vi "Signalgenerator (2).vi"() -> ()   [LabVIEW 2013]
panel:
  in  "Set Phase":bool
  in  "Phase":dbl
  in  "Set Offset":bool
  in  "Offset":dbl
  in  "Set Amplitude":bool
  in  "Amplitude":dbl
  in  "Set Frequency":bool
  in  "Frequency":dbl
  in  "Waveform":T1(radio)
  in  "Display Mode":T2(radio)
  in  "Read":bool
  in  "Write":bool
  in  "Exit":bool
  in  "Connect":bool
  in  "VISA Address":refnum<visa-resource-name>
  out "Return":string
  in  "Command":string
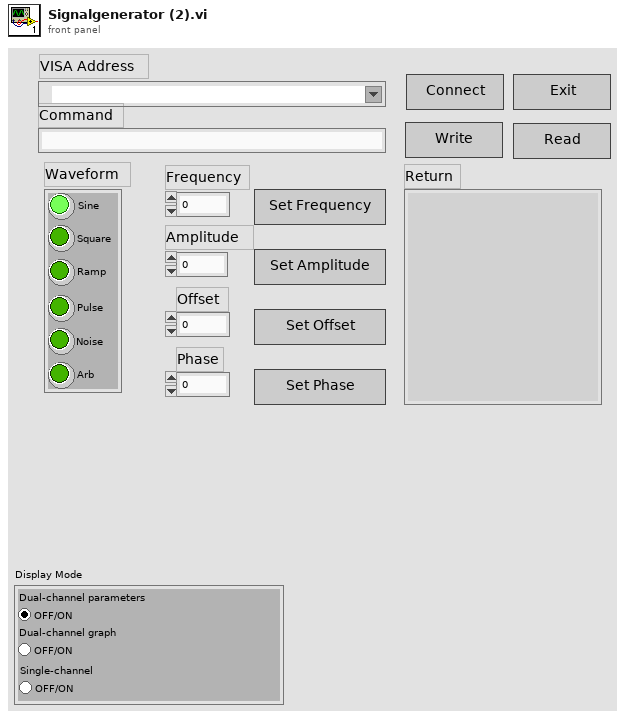
[diagram p1: front panel]
types:
  T1 = enum32{"Sine", "Square", "Ramp", "Pulse", "Noise", "Arb"}
  T2 = enum32{"Dual-channel parameters", "Dual-channel graph", "Single-channel"}
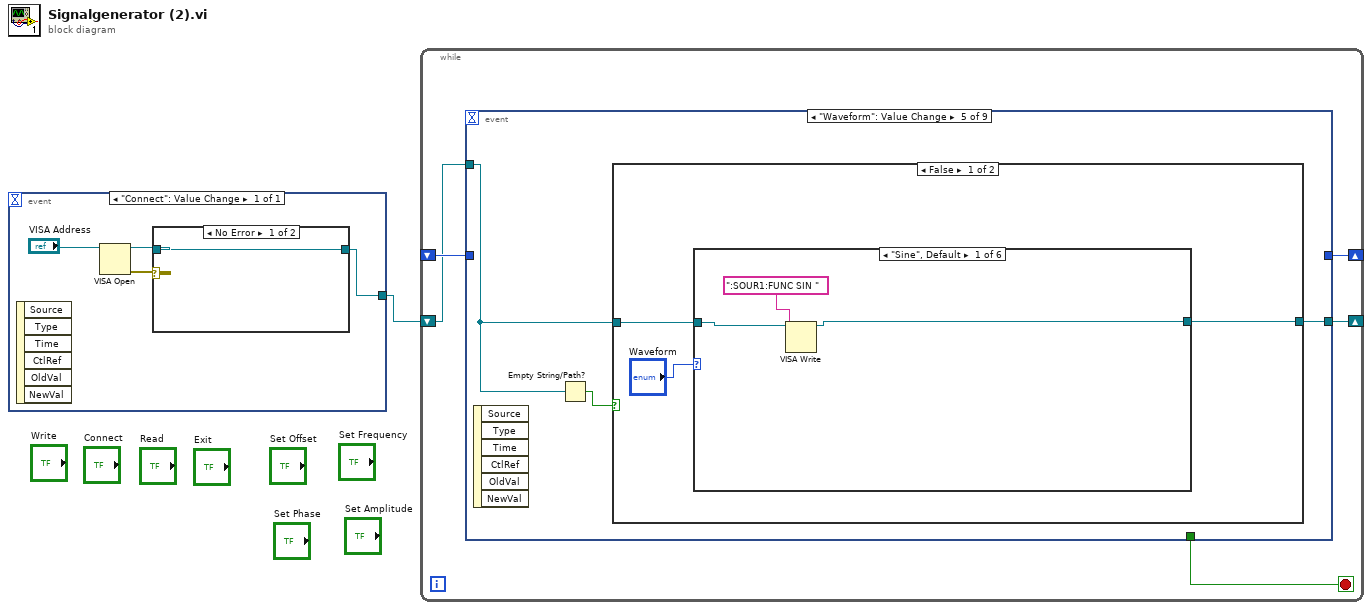
[diagram p0: block diagram]
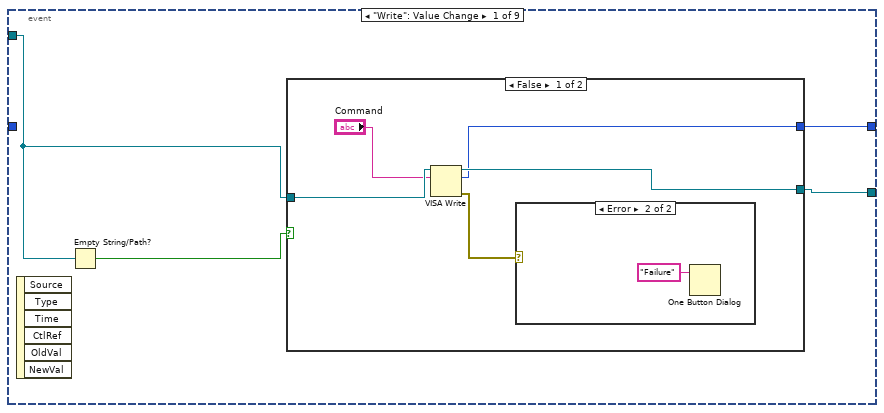
[diagram p2: hidden frame]
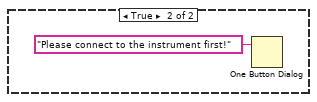
[diagram p4: hidden frame]
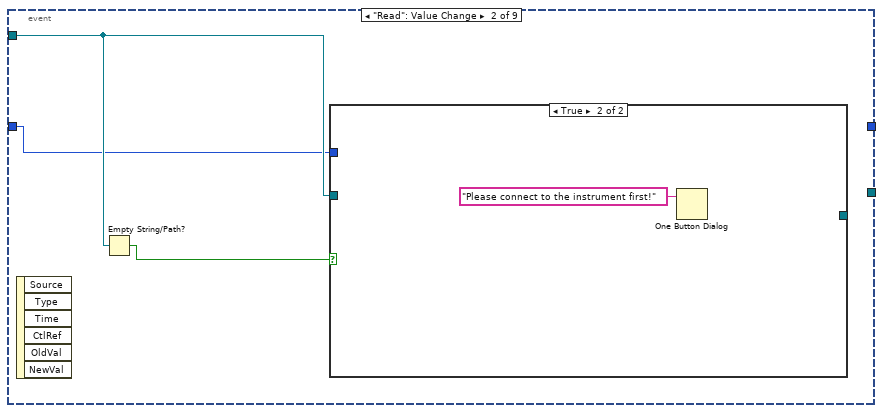
[diagram p5: hidden frame]
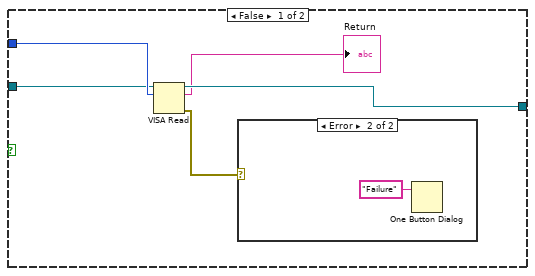
[diagram p6: hidden frame]
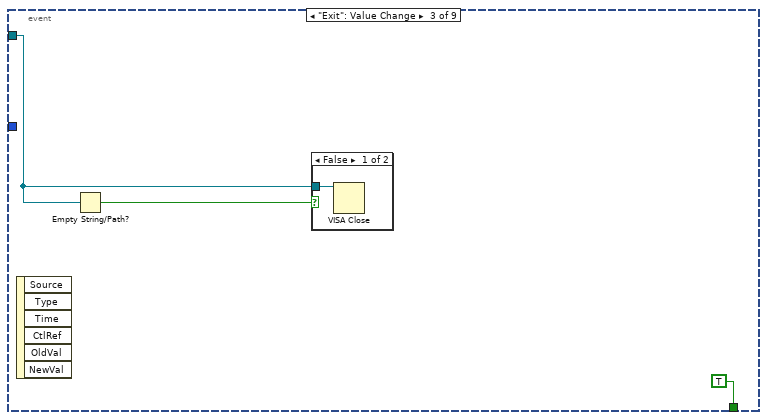
[diagram p8: hidden frame]
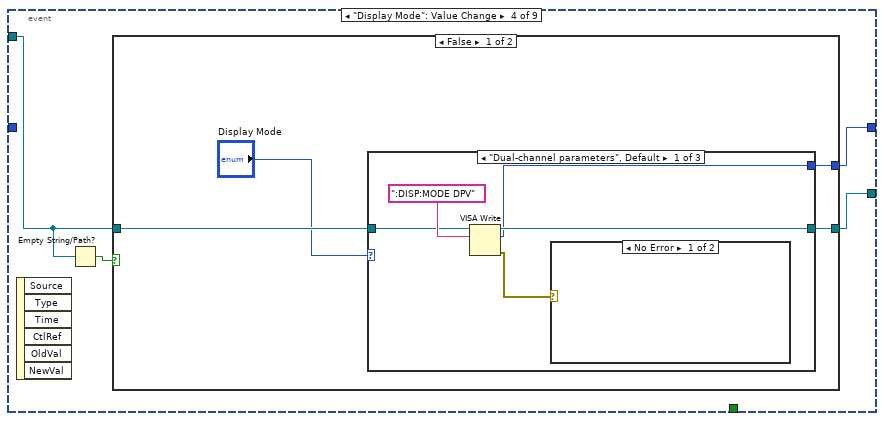
[diagram p10: hidden frame]
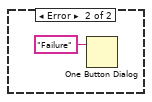
[diagram p11: hidden frame]
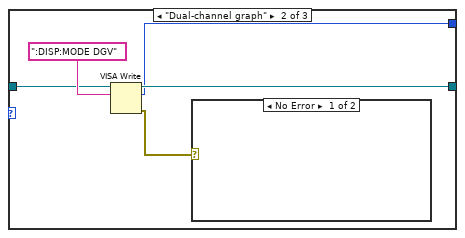
[diagram p12: hidden frame]
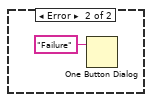
[diagram p13: hidden frame]
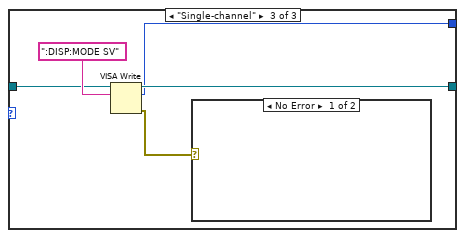
[diagram p14: hidden frame]
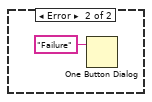
[diagram p15: hidden frame]
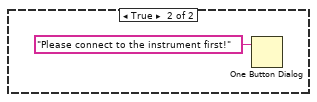
[diagram p16: hidden frame]
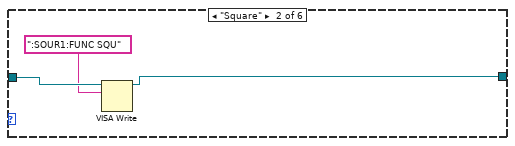
[diagram p17: hidden frame]
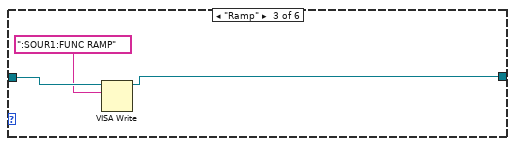
[diagram p18: hidden frame]
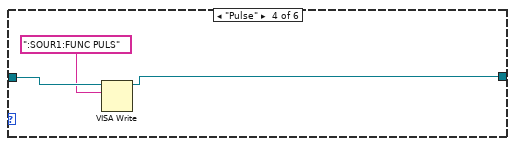
[diagram p19: hidden frame]
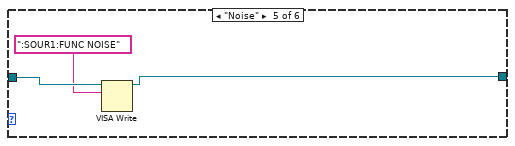
[diagram p20: hidden frame]
diagram:
  n1 = event shown="[0] \"Connect\": Value Change" {
    selector: _ -> [_]
    dyn-events: _ -> [_]
    timeout: _ -> [_]
    tunnel: [w3] -> w1
    event "Connect": Value Change {
      n2 = event-data() -> ()  [unwired: 1 in, 6 out]
      n3 = VISA Open(VISA resource name="VISA Address") -> (VISA resource name=w4:refnum<visa-resource-name>, error out=w5:errorcluster)  [unwired: 4 in]
      n4 = case shown="No Error" w5 {
        tunnel: w4 -> [w6 _]
        tunnel: [w6 _] -> w3
        frame No Error {
        }
        frame Error {
          n5 = One Button Dialog(message="Connect failed!\nInvalid address!") -> ()  [unwired: 1 in, 1 out]
        }
      }
    }
  }
  n6 = while {
    shift-right: [w10] -> _
    shift-left: w1 -> [w11]
    shift-right: [w9] -> _
    shift-left: _ -> [w12]
    stop <- w8 stop-if-true
    n7 = event shown="[4] \"Waveform\": Value Change" {
      selector: _ -> [_ _ _ _ _ _ _ _ _]
      dyn-events: _ -> [_ _ _ _ _ _ _ _ _]
      timeout: _ -> [_ _ _ _ _ _ _ _ _]
      tunnel: w12 -> [_ w24 _ _ _ _ _ _ _]
      tunnel: w11 -> [w15 w25 w35 w38 w66 w92 w105 w120 w134]
      tunnel: [w14 _ _ w40 w65 w90 w103 w117 w131] -> w10
      tunnel: [w13 _ _ w41 _ w91 w104 w118 w132] -> w9
      tunnel: [_ _ TRUE _ _ _ _ _ _] -> w8
      event "Write": Value Change {
        n8 = event-data() -> ()  [unwired: 1 in, 6 out]
        n9 = Empty String/Path?(string/path=w15) -> (empty?=w16:bool)
        n10 = case shown="False" w16 {
          tunnel: [w20 _] -> w14
          tunnel: [w19 _] -> w13
          tunnel: w15 -> [w18 _]
          frame False {
            n11 = VISA Write(VISA resource name=w18, write buffer="Command") -> (VISA resource name out=w20:refnum<visa-resource-name>, return count=w19:u32, error out=w21:errorcluster)  [unwired: 1 in]
            n12 = case shown="Error" w21 {
              frame No Error {
              }
              frame Error {
                n13 = One Button Dialog(message="Failure") -> ()  [unwired: 1 in, 1 out]
              }
            }
          }
          frame True {
            n14 = One Button Dialog(message="Please connect to the instrument first!") -> ()  [unwired: 1 in, 1 out]
          }
        }
      }
      event "Read": Value Change {
        n15 = event-data() -> ()  [unwired: 1 in, 6 out]
        n16 = Empty String/Path?(string/path=w25) -> (empty?=w26:bool)
        n17 = case shown="True" w26 {
          tunnel: [w31 _] -> _
          tunnel: w24 -> [w29 _]
          tunnel: w25 -> [w28 _]
          frame False {
            n18 = VISA Read(VISA resource name=w28, byte count=w29) -> (VISA resource name out=w31:refnum<visa-resource-name>, read buffer=→"Return":string, error out=w30:errorcluster)  [unwired: 1 in, 1 out]
            n19 = case shown="Error" w30 {
              frame No Error {
              }
              frame Error {
                n20 = One Button Dialog(message="Failure") -> ()  [unwired: 1 in, 1 out]
              }
            }
          }
          frame True {
            n21 = One Button Dialog(message="Please connect to the instrument first!") -> ()  [unwired: 1 in, 1 out]
          }
        }
      }
      event "Exit": Value Change {
        n22 = event-data() -> ()  [unwired: 1 in, 6 out]
        n23 = Empty String/Path?(string/path=w35) -> (empty?=w36:bool)
        n24 = case shown="False" w36 {
          tunnel: w35 -> [w37 _]
          frame False {
            n25 = VISA Close(VISA resource name=w37) -> ()  [unwired: 1 in, 1 out]
          }
          frame True {
          }
        }
      }
      event "Display Mode": Value Change {
        n26 = event-data() -> ()  [unwired: 1 in, 6 out]
        n27 = Empty String/Path?(string/path=w38) -> (empty?=w39:bool)
        n28 = case shown="False" w39 {
          tunnel: [w45 _] -> w40
          tunnel: [w44 _] -> w41
          tunnel: w38 -> [w43 _]
          frame False {
            n29 = case shown="\"Dual-channel parameters\", Default" "Display Mode" {
              tunnel: [w48 w54 w60] -> w45
              tunnel: [w47 w53 w59] -> w44
              tunnel: w43 -> [w46 w52 w58]
              frame "Dual-channel parameters", Default {
                n30 = VISA Write(VISA resource name=w46, write buffer=":DISP:MODE DPV" ("Command 2")) -> (VISA resource name out=w48:refnum<visa-resource-name>, return count=w47:u32, error out=w49:errorcluster)  [unwired: 1 in]
                n31 = case shown="No Error" w49 {
                  frame No Error {
                  }
                  frame Error {
                    n32 = One Button Dialog(message="Failure") -> ()  [unwired: 1 in, 1 out]
                  }
                }
              }
              frame "Dual-channel graph" {
                n33 = VISA Write(VISA resource name=w52, write buffer=":DISP:MODE DGV" ("Command 2")) -> (VISA resource name out=w54:refnum<visa-resource-name>, return count=w53:u32, error out=w55:errorcluster)  [unwired: 1 in]
                n34 = case shown="No Error" w55 {
                  frame No Error {
                  }
                  frame Error {
                    n35 = One Button Dialog(message="Failure") -> ()  [unwired: 1 in, 1 out]
                  }
                }
              }
              frame "Single-channel" {
                n36 = VISA Write(VISA resource name=w58, write buffer=":DISP:MODE SV" ("Command 2")) -> (VISA resource name out=w60:refnum<visa-resource-name>, return count=w59:u32, error out=w61:errorcluster)  [unwired: 1 in]
                n37 = case shown="No Error" w61 {
                  frame No Error {
                  }
                  frame Error {
                    n38 = One Button Dialog(message="Failure") -> ()  [unwired: 1 in, 1 out]
                  }
                }
              }
            }
          }
          frame True {
            n39 = One Button Dialog(message="Please connect to the instrument first!") -> ()  [unwired: 1 in, 1 out]
          }
        }
      }
      event "Waveform": Value Change {
        n40 = event-data() -> ()  [unwired: 1 in, 6 out]
        n41 = Empty String/Path?(string/path=w66) -> (empty?=w67:bool)
        n42 = case shown="False" w67 {
          tunnel: w66 -> [w69 _]
          tunnel: [w68 _] -> w65
          frame False {
            n43 = case shown="\"Sine\", Default" "Waveform" {
              tunnel: w69 -> [w72 w76 w79 w82 w85 w88]
              tunnel: [w71 w74 w77 w80 w83 w86] -> w68
              frame "Sine", Default {
                n44 = VISA Write(VISA resource name=w72, write buffer=":SOUR1:FUNC SIN ") -> (VISA resource name out=w71:refnum<visa-resource-name>)  [unwired: 1 in, 2 out]
              }
              frame "Square" {
                n45 = VISA Write(VISA resource name=w76, write buffer=":SOUR1:FUNC SQU") -> (VISA resource name out=w74:refnum<visa-resource-name>)  [unwired: 1 in, 2 out]
              }
              frame "Ramp" {
                n46 = VISA Write(VISA resource name=w79, write buffer=":SOUR1:FUNC RAMP") -> (VISA resource name out=w77:refnum<visa-resource-name>)  [unwired: 1 in, 2 out]
              }
              frame "Pulse" {
                n47 = VISA Write(VISA resource name=w82, write buffer=":SOUR1:FUNC PULS") -> (VISA resource name out=w80:refnum<visa-resource-name>)  [unwired: 1 in, 2 out]
              }
              frame "Noise" {
                n48 = VISA Write(VISA resource name=w85, write buffer=":SOUR1:FUNC NOISE") -> (VISA resource name out=w83:refnum<visa-resource-name>)  [unwired: 1 in, 2 out]
              }
              frame "Arb" {
                n49 = VISA Write(VISA resource name=w88, write buffer=":SOUR1:APPL:ARB") -> (VISA resource name out=w86:refnum<visa-resource-name>)  [unwired: 1 in, 2 out]
              }
            }
          }
          frame True {
            n50 = One Button Dialog(message="Please connect to the instrument first!") -> ()  [unwired: 1 in, 1 out]
          }
        }
      }
      event "Set Frequency": Value Change {
        n51 = event-data() -> ()  [unwired: 1 in, 6 out]
        n52 = Empty String/Path?(string/path=w92) -> (empty?=w93:bool)
        n53 = case shown="False" w93 {
          tunnel: w92 -> [w100 _]
          tunnel: [w99 _] -> w91
          tunnel: [w98 _] -> w90
          frame False {
            n54 = Format Into String(format string="%.; :SOUR1:FREQ %5.3f", "Frequency") -> (resulting string=w94:string)  [unwired: 2 in, 1 out]
            n55 = VISA Write(VISA resource name=w100, write buffer=w94) -> (VISA resource name out=w98:refnum<visa-resource-name>, return count=w99:u32, error out=w97:errorcluster)  [unwired: 1 in]
            n56 = case shown="No Error" w97 {
              frame No Error {
              }
              frame Error {
                n57 = One Button Dialog(message="Failure") -> ()  [unwired: 1 in, 1 out]
              }
            }
          }
          frame True {
            n58 = One Button Dialog(message="Please connect to the instrument first!") -> ()  [unwired: 1 in, 1 out]
          }
        }
      }
      event "Set Amplitude": Value Change {
        n59 = event-data() -> ()  [unwired: 1 in, 6 out]
        n60 = Empty String/Path?(string/path=w105) -> (empty?=w106:bool)
        n61 = case shown="False" w106 {
          tunnel: w105 -> [w114 _]
          tunnel: [w113 _] -> w104
          tunnel: [w112 _] -> w103
          frame False {
            n62 = Format Into String(format string="%.; :SOUR1:VOLT %5.3f", "Amplitude") -> (resulting string=w110:string, error out=w108:errorcluster)  [unwired: 2 in]
            n63 = VISA Write(VISA resource name=w114, write buffer=w110, error in (no error)=w108) -> (VISA resource name out=w112:refnum<visa-resource-name>, return count=w113:u32, error out=w111:errorcluster)
            n64 = case shown="No Error" w111 {
              frame No Error {
              }
              frame Error {
                n65 = One Button Dialog(message="Failure") -> ()  [unwired: 1 in, 1 out]
              }
            }
          }
          frame True {
            n66 = One Button Dialog(message="Please connect to the instrument first!") -> ()  [unwired: 1 in, 1 out]
          }
        }
      }
      event "Set Offset": Value Change {
        n67 = event-data() -> ()  [unwired: 1 in, 6 out]
        n68 = Empty String/Path?(string/path=w120) -> (empty?=w119:bool)
        n69 = case shown="False" w119 {
          tunnel: w120 -> [w128 _]
          tunnel: [w127 _] -> w118
          tunnel: [w126 _] -> w117
          frame False {
            n70 = Format Into String(format string="%.; :SOUR1:VOLT:OFFS %5.3f", "Offset") -> (resulting string=w124:string, error out=w122:errorcluster)  [unwired: 2 in]
            n71 = VISA Write(VISA resource name=w128, write buffer=w124, error in (no error)=w122) -> (VISA resource name out=w126:refnum<visa-resource-name>, return count=w127:u32, error out=w125:errorcluster)
            n72 = case shown="No Error" w125 {
              frame No Error {
              }
              frame Error {
                n73 = One Button Dialog(message="Failure") -> ()  [unwired: 1 in, 1 out]
              }
            }
          }
          frame True {
            n74 = One Button Dialog(message="Please connect to the instrument first!") -> ()  [unwired: 1 in, 1 out]
          }
        }
      }
      event "Set Phase": Value Change {
        n75 = event-data() -> ()  [unwired: 1 in, 6 out]
        n76 = Empty String/Path?(string/path=w134) -> (empty?=w133:bool)
        n77 = case shown="False" w133 {
          tunnel: w134 -> [w142 _]
          tunnel: [w141 _] -> w132
          tunnel: [w140 _] -> w131
          frame False {
            n78 = Format Into String(format string="%.; :SOUR1:PHAS %5.3f", "Phase") -> (resulting string=w138:string, error out=w136:errorcluster)  [unwired: 2 in]
            n79 = VISA Write(VISA resource name=w142, write buffer=w138, error in (no error)=w136) -> (VISA resource name out=w140:refnum<visa-resource-name>, return count=w141:u32, error out=w139:errorcluster)
            n80 = case shown="No Error" w139 {
              frame No Error {
              }
              frame Error {
                n81 = One Button Dialog(message="Failure") -> ()  [unwired: 1 in, 1 out]
              }
            }
          }
          frame True {
            n82 = One Button Dialog(message="Please connect to the instrument first!") -> ()  [unwired: 1 in, 1 out]
          }
        }
      }
    }
  }
